vi "xy to angle.vi"(9 "x":dbl, 10 "y":dbl) -> (1 "red angle":dbl, 2 "Blue angle":dbl)   [LabVIEW 2020]
uses:
  Robot Global Data.vi
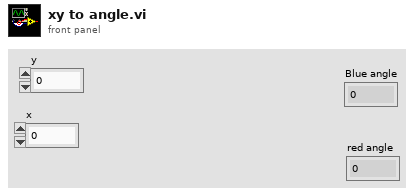
[diagram p1: front panel]
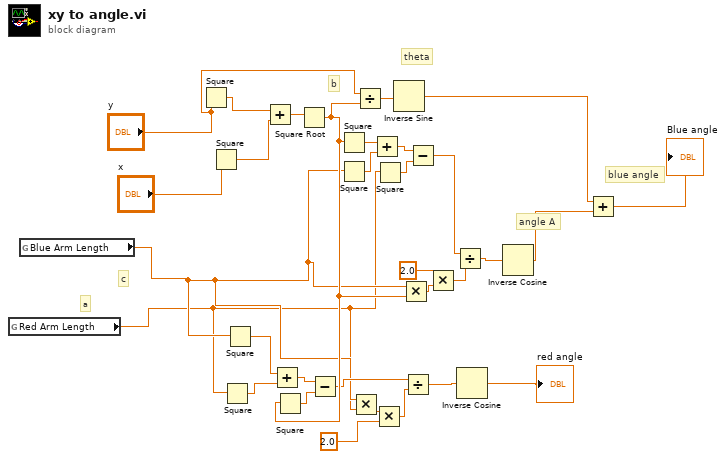
[diagram p0: block diagram]
diagram:
  # "blue angle"
  # "angle A"
  # "a"
  # "c"
  # "theta"
  # "b"
  n1 = global read "Robot Global Data.vi" "Red Arm Length"() -> (w1:dbl)
  n2 = global read "Robot Global Data.vi" "Blue Arm Length"() -> (w2:dbl)
  n3 = Square(x="y") -> (x^2=w29:dbl)
  n4 = Square(x="x") -> (x^2=w31:dbl)
  n5 = Square(x=w1) -> (x^2=w10:dbl)
  n6 = Square(x=w2) -> (x^2=w11:dbl)
  n7 = Add(x=w29, y=w31) -> (x+y=w28:dbl)
  n8 = Add(x=w11, y=w10) -> (x+y=w13:dbl)
  n9 = Square Root(x=w28) -> (sqrt(x)=w9:dbl)
  n10 = Square(x=w9) -> (x^2=w12:dbl)
  n11 = Subtract(x=w13, y=w12) -> (x-y=w8:dbl)
  n12 = Square(x=w9) -> (x^2=w24:dbl)
  n13 = Square(x=w2) -> (x^2=w23:dbl)
  n14 = Multiply(x=w2, y=w1) -> (x*y=w7:dbl)
  n15 = Divide(x="y", y=w9) -> (x/y=w26:dbl)
  n16 = Add(x=w24, y=w23) -> (x+y=w25:dbl)
  n17 = Multiply(x=w7, y=2.0) -> (x*y=w5:dbl)
  n18 = Square(x=w1) -> (x^2=w22:dbl)
  n19 = Inverse Sine(1:w26) -> (0:w15:dbl)
  n20 = Multiply(x=w2, y=w9) -> (x*y=w20:dbl)
  n21 = Divide(x=w8, y=w5) -> (x/y=w4:dbl)
  n22 = Subtract(x=w25, y=w22) -> (x-y=w21:dbl)
  n23 = Multiply(x=2.0, y=w20) -> (x*y=w19:dbl)
  n24 = Divide(x=w21, y=w19) -> (x/y=w17:dbl)
  n25 = Inverse Cosine(1:w4) -> (0:→"red angle":dbl)
  n26 = Inverse Cosine(1:w17) -> (0:w16:dbl)
  n27 = Add(x=w15, y=w16) -> (x+y=→"Blue angle":dbl)
